vi "ReadPhysicsSettings.vi"   [LabVIEW 2020]
uses:
  <vilib>/Utility/config.llb/Read Key (Double).vi
  SettingVariable.vi
  <vilib>/Utility/config.llb/NI_LVConfig.lvlib
types:
  T1 = typedef "NI_LVConfig.lvlib/Config Data RefNum.ctl" = refnum<k1>
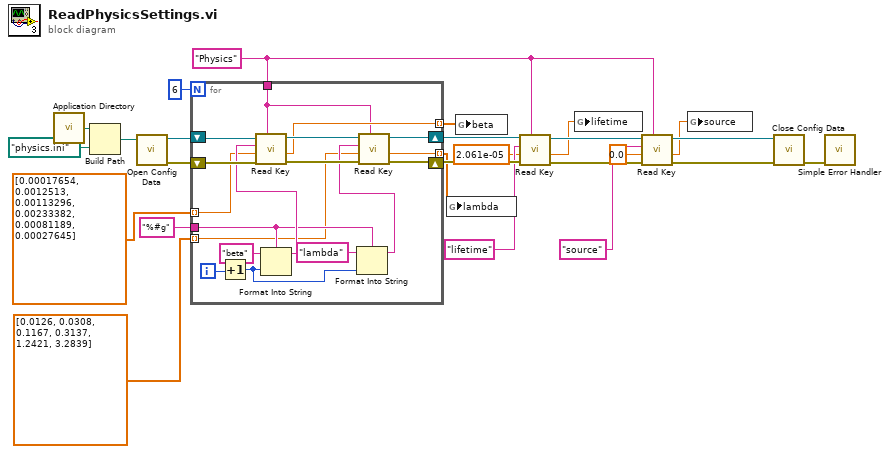
[diagram p0: block diagram]
diagram:
  w6 = "Physics"
  n1 = call <vilib>:"Application Directory.vi"() -> ("Application Directory"=w24:path)
  n2 = Build Path(base path=w24, name or relative path=path "physics.ini") -> (appended path=w23:path)
  n3 = call <vilib>:"Open Config Data.vi"("configuration file path"=w23) -> ("error out"=w20:errorcluster, "refnum"=w21:T1)  [unwired: 8 in, 1 out]
  n4 = for {
    N: 6 -> [_]
    tunnel: [w33] -> w17 mode=indexing
    tunnel: [w32] -> w16 mode=indexing
    shift-right: [w31] -> w18
    shift-left: w20 -> [w42]
    shift-right: [w30] -> w15
    shift-left: w21 -> [w43]
    tunnel: w6 -> [w29]
    tunnel: "%#g" ("format string") -> [w28]
    tunnel: dbl[] [0.00017654, 0.0012513, 0.00113296, 0.00233382, 0.00081189, 0.00027645] -> [w27] mode=indexing
    tunnel: dbl[] [0.0126, 0.0308, 0.1167, 0.3137, 1.2421, 3.2839] -> [w26] mode=indexing
    i -> [w39]
    n5 = Increment(x=w39) -> (x+1=w36:i32)
    n6 = Format Into String(format string=w28, initial string="beta", w36) -> (resulting string=w37:string)  [unwired: 1 in, 1 out]
    n7 = call-poly <vilib>:"Read Key.vi"("section"=w29, "error in (no error)"=w42, "default value"=w27, "key"=w37, "refnum"=w43) -> ("error out"=w40:errorcluster, "value"=w33:dbl, "refnum out"=w41:T1)  [unwired: 3 in, 1 out]
    n8 = Format Into String(format string=w28, initial string="lambda", w36) -> (resulting string=w34:string)  [unwired: 1 in, 1 out]
    n9 = call-poly <vilib>:"Read Key.vi"("section"=w29, "error in (no error)"=w40, "default value"=w26, "key"=w34, "refnum"=w41) -> ("error out"=w31:errorcluster, "value"=w32:dbl, "refnum out"=w30:T1)  [unwired: 3 in, 1 out]
  }
  n10 = global write "SettingVariable.vi" "lambda"(w16) -> ()
  n11 = global write "SettingVariable.vi" "beta"(w17) -> ()
  n12 = call-poly <vilib>:"Read Key.vi"("section"=w6, "error in (no error)"=w18, "default value"=2.061e-05, "key"="lifetime" ("initial string"), "refnum"=w15) -> ("error out"=w12:errorcluster, "value"=w8:dbl, "refnum out"=w13:T1)  [unwired: 3 in, 1 out]
  n13 = global write "SettingVariable.vi" "lifetime"(w8) -> ()
  n14 = call-poly <vilib>:"Read Key.vi"("section"=w6, "error in (no error)"=w12, "default value"=0.0, "key"="source" ("initial string"), "refnum"=w13) -> ("error out"=w10:errorcluster, "value"=w7:dbl, "refnum out"=w9:T1)  [unwired: 3 in, 1 out]
  n15 = global write "SettingVariable.vi" "source"(w7) -> ()
  n16 = call <vilib>:"Close Config Data.vi"("error in (no error)"=w10, "refnum"=w9) -> ("error out"=w19:errorcluster)  [unwired: 8 in, 1 out]
  n17 = call <vilib>:"Simple Error Handler.vi"("error in (no error)"=w19) -> ()  [unwired: 1 in, 8 out]
